vi "INIT.vi"(8 "error in (no error)":errorcluster, 11 "Control-Server in":refnum<class "Control-Server.lvclass">) -> (0 "error out":errorcluster, 3 "Control-Server out":refnum<class "Control-Server.lvclass">)   [LabVIEW 2018, in "Control-Server.lvclass"]
uses:
  Control-Server.lvclass
  Config/config_names_def.ctl
  Config/Config.lvclass
  Control-Server.lvclass/Control-Server.ctl
  dependecies/globalVarII.vi
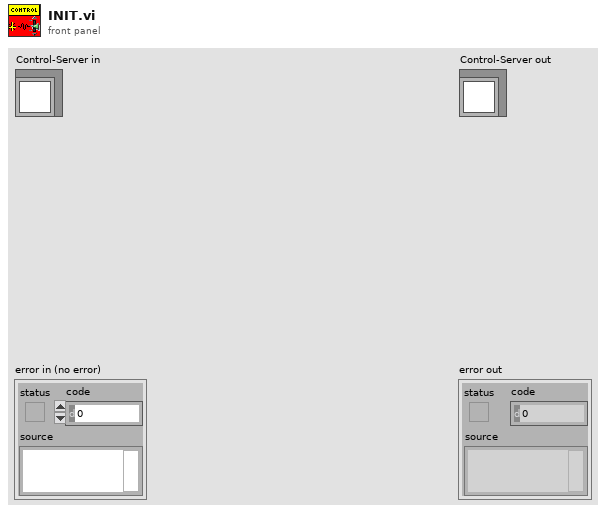
[diagram p1: front panel]
types:
  T1 = typedef "Config.lvclass/config_names_def.ctl" = string
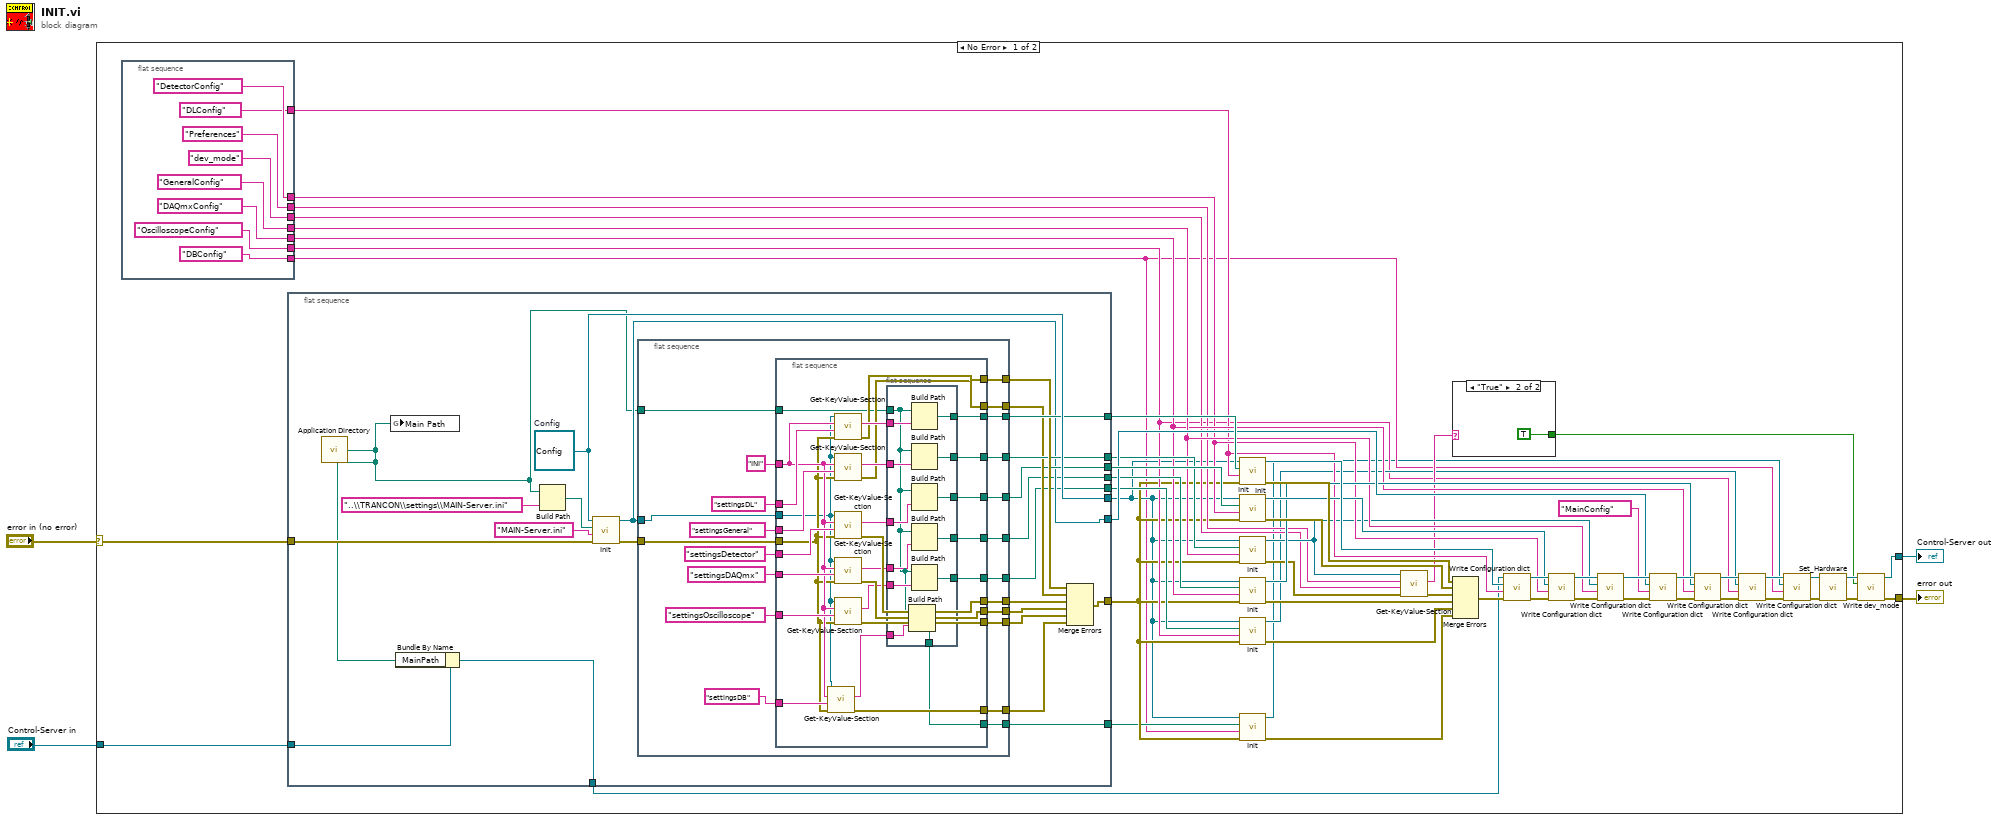
[diagram p0: block diagram]
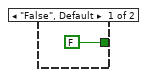
[diagram p2: hidden frame]
diagram:
  n1 = case shown="No Error" "error in (no error)" {
    selector: "error in (no error)" -> [w56 w157]
    tunnel: [w23 w157] -> w3
    tunnel: [w24 w156] -> w4
    tunnel: "Control-Server in" -> [w6 w156]
    frame No Error {
      n2 = flat-sequence {
        tunnel: [T1 "GeneralConfig" ("Combo Box")] -> w38
        tunnel: [T1 "DAQmxConfig" ("Combo Box")] -> w37
        tunnel: [T1 "DetectorConfig" ("Combo Box")] -> w36
        tunnel: [T1 "DLConfig" ("Combo Box")] -> w35
        tunnel: ["Preferences" ("Section")] -> w28
        tunnel: ["dev_mode" ("Key")] -> w27
        tunnel: [T1 "OscilloscopeConfig" ("Combo Box")] -> w18
        tunnel: [T1 "DBConfig" ("Combo Box")] -> w8
        frame #0 {
        }
      }
      n3 = flat-sequence {
        tunnel: [w91] -> w10
        tunnel: [w88] -> w57
        tunnel: [w86] -> w42
        tunnel: w56 -> [w82]
        tunnel: [w81] -> w12
        tunnel: [w80] -> w55
        tunnel: [w79] -> w45
        tunnel: [w77] -> w41
        tunnel: [w76] -> w21
        tunnel: [w73] -> w9
        tunnel: w6 -> [w72]
        tunnel: [w70] -> w5
        frame #0 {
          w91 = refnum<class "Config.lvclass"> refnum  # Config
          n4 = call <vilib>:"Application Directory.vi"() -> ("Application Directory"=w71:path)
          n5 = global write "globalVarII.vi" "Main Path"(w71) -> ()
          n6 = Bundle By Name(cluster=w72, "MainPath"=w71) -> (w70:refnum<class "Control-Server.lvclass">)
          n7 = Build Path(base path=w71, name or relative path="..\\TRANCON\\settings\\MAIN-Server.ini" ("nom ou chemin relatif")) -> (appended path=w90:path)
          n8 = call "Init.vi"("error in"=w82, "Name"="MAIN-Server.ini", "Path"=w90, "Config in"=w91) -> ("error out"=w85:errorcluster, "Config out"=w79:refnum<class "Config.lvclass">)  [unwired: 6 in]
          n9 = flat-sequence {
            tunnel: [w113] -> w88
            tunnel: [w111] -> w87
            tunnel: [w110] -> w86
            tunnel: w79 -> [w109]
            tunnel: w85 -> [w106]
            tunnel: [w105] -> w84
            tunnel: [w104] -> w83
            tunnel: w71 -> [w103]
            tunnel: [w102] -> w80
            tunnel: [w100] -> w78
            tunnel: [w99] -> w77
            tunnel: [w97] -> w76
            tunnel: [w96] -> w75
            tunnel: [w94] -> w74
            tunnel: [w93] -> w73
            frame #0 {
              n10 = flat-sequence {
                tunnel: "settingsDL" ("Key") -> [w142]
                tunnel: [w140] -> w113
                tunnel: "settingsGeneral" ("Key") -> [w139]
                tunnel: [w138] -> w111
                tunnel: [w136] -> w110
                tunnel: w109 -> [w116]
                tunnel: "INI" ("Section") -> [w120]
                tunnel: "settingsDetector" ("Key") -> [w135]
                tunnel: w106 -> [w118]
                tunnel: [w134] -> w105
                tunnel: [w133] -> w104
                tunnel: w103 -> [w127]
                tunnel: [w131] -> w102
                tunnel: "settingsDAQmx" ("Key") -> [w130]
                tunnel: [w129] -> w100
                tunnel: [w126] -> w99
                tunnel: "settingsOscilloscope" ("Key") -> [w125]
                tunnel: [w123] -> w97
                tunnel: [w122] -> w96
                tunnel: "settingsDB" ("Key") -> [w121]
                tunnel: [w117] -> w94
                tunnel: [w115] -> w93
                frame #0 {
                  n11 = call-dynamic "Get-KeyValue-Section.vi"("error in (no error)"=w118, "Key"=w121, "Section"=w120, "Config in"=w116) -> ("error out"=w117:errorcluster, "Value"=w119:string)  [unwired: 5 in, 1 out]
                  n12 = call-dynamic "Get-KeyValue-Section.vi"("error in (no error)"=w118, "Key"=w142, "Section"=w120, "Config in"=w116) -> ("error out"=w138:errorcluster, "Value"=w141:string)  [unwired: 5 in, 1 out]
                  n13 = call-dynamic "Get-KeyValue-Section.vi"("error in (no error)"=w118, "Key"=w139, "Section"=w120, "Config in"=w116) -> ("error out"=w134:errorcluster, "Value"=w137:string)  [unwired: 5 in, 1 out]
                  n14 = call-dynamic "Get-KeyValue-Section.vi"("error in (no error)"=w118, "Key"=w135, "Section"=w120, "Config in"=w116) -> ("error out"=w133:errorcluster, "Value"=w132:string)  [unwired: 5 in, 1 out]
                  n15 = call-dynamic "Get-KeyValue-Section.vi"("error in (no error)"=w118, "Key"=w130, "Section"=w120, "Config in"=w116) -> ("error out"=w129:errorcluster, "Value"=w128:string)  [unwired: 5 in, 1 out]
                  n16 = call-dynamic "Get-KeyValue-Section.vi"("error in (no error)"=w118, "Key"=w125, "Section"=w120, "Config in"=w116) -> ("error out"=w122:errorcluster, "Value"=w124:string)  [unwired: 5 in, 1 out]
                  n17 = flat-sequence {
                    tunnel: w141 -> [w155]
                    tunnel: [w154] -> w140
                    tunnel: w137 -> [w153]
                    tunnel: [w152] -> w136
                    tunnel: w132 -> [w151]
                    tunnel: [w150] -> w131
                    tunnel: w128 -> [w149]
                    tunnel: w127 -> [w144]
                    tunnel: [w148] -> w126
                    tunnel: w124 -> [w147]
                    tunnel: [w146] -> w123
                    tunnel: w119 -> [w145]
                    tunnel: [w143] -> w115
                    frame #0 {
                      n18 = Build Path(base path=w144, name or relative path=w145) -> (appended path=w143:path)
                      n19 = Build Path(base path=w144, name or relative path=w155) -> (appended path=w154:path)
                      n20 = Build Path(base path=w144, name or relative path=w153) -> (appended path=w152:path)
                      n21 = Build Path(base path=w144, name or relative path=w151) -> (appended path=w150:path)
                      n22 = Build Path(base path=w144, name or relative path=w149) -> (appended path=w148:path)
                      n23 = Build Path(base path=w144, name or relative path=w147) -> (appended path=w146:path)
                    }
                  }
                }
              }
            }
          }
          n24 = Merge Errors(w87, w84, w83, w78, w75, w74) -> (w81:errorcluster)
        }
      }
      n25 = call "Init.vi"("error in"=w12, "Name"=w35, "Path"=w57, "Config in"=w10) -> ("error out"=w59:errorcluster, "Config out"=w54:refnum<class "Config.lvclass">)  [unwired: 6 in]
      n26 = call "Init.vi"("error in"=w12, "Name"=w36, "Path"=w55, "Config in"=w10) -> ("error out"=w58:errorcluster, "Config out"=w51:refnum<class "Config.lvclass">)  [unwired: 6 in]
      n27 = call "Init.vi"("error in"=w12, "Name"=w38, "Path"=w42, "Config in"=w10) -> ("error out"=w31:errorcluster, "Config out"=w29:refnum<class "Config.lvclass">)  [unwired: 6 in]
      n28 = call "Init.vi"("error in"=w12, "Name"=w37, "Path"=w41, "Config in"=w10) -> ("error out"=w39:errorcluster, "Config out"=w40:refnum<class "Config.lvclass">)  [unwired: 6 in]
      n29 = call "Init.vi"("error in"=w12, "Name"=w18, "Path"=w21, "Config in"=w10) -> ("error out"=w22:errorcluster, "Config out"=w19:refnum<class "Config.lvclass">)  [unwired: 6 in]
      n30 = call "Init.vi"("error in"=w12, "Name"=w8, "Path"=w9, "Config in"=w10) -> ("error out"=w11:errorcluster, "Config out"=w7:refnum<class "Config.lvclass">)  [unwired: 6 in]
      n31 = call-dynamic "Get-KeyValue-Section.vi"("error in (no error)"=w31, "Key"=w27, "Section"=w28, "Config in"=w29) -> ("error out"=w30:errorcluster, "Value"=w26:string)  [unwired: 5 in, 1 out]
      n32 = case shown="\"True\"" w26 {
        tunnel: [FALSE TRUE] -> w25
        frame "False", Default {
        }
        frame "True" {
        }
      }
      n33 = Merge Errors(w59, w58, w30, w39, w22, w11) -> (w49:errorcluster)
      n34 = call "Write Configuration dict.vi"("error in (no error)"=w49, "Config Name"=w35, "Config.lvclass"=w54, "Control in"=w5) -> ("error out"=w52:errorcluster, "Control out"=w53:refnum<class "Control-Server.lvclass">)  [unwired: 6 in]
      n35 = call "Write Configuration dict.vi"("error in (no error)"=w52, "Config Name"=w36, "Config.lvclass"=w51, "Control in"=w53) -> ("error out"=w48:errorcluster, "Control out"=w50:refnum<class "Control-Server.lvclass">)  [unwired: 6 in]
      n36 = call "Write Configuration dict.vi"("error in (no error)"=w48, "Config Name"=w38, "Config.lvclass"=w29, "Control in"=w50) -> ("error out"=w47:errorcluster, "Control out"=w46:refnum<class "Control-Server.lvclass">)  [unwired: 6 in]
      n37 = call "Write Configuration dict.vi"("error in (no error)"=w47, "Config Name"=T1 "MainConfig" ("Combo Box"), "Config.lvclass"=w45, "Control in"=w46) -> ("error out"=w43:errorcluster, "Control out"=w44:refnum<class "Control-Server.lvclass">)  [unwired: 6 in]
      n38 = call "Write Configuration dict.vi"("error in (no error)"=w43, "Config Name"=w37, "Config.lvclass"=w40, "Control in"=w44) -> ("error out"=w17:errorcluster, "Control out"=w20:refnum<class "Control-Server.lvclass">)  [unwired: 6 in]
      n39 = call "Write Configuration dict.vi"("error in (no error)"=w17, "Config Name"=w18, "Config.lvclass"=w19, "Control in"=w20) -> ("error out"=w16:errorcluster, "Control out"=w13:refnum<class "Control-Server.lvclass">)  [unwired: 6 in]
      n40 = call "Write Configuration dict.vi"("error in (no error)"=w16, "Config Name"=w8, "Config.lvclass"=w7, "Control in"=w13) -> ("error out"=w15:errorcluster, "Control out"=w14:refnum<class "Control-Server.lvclass">)  [unwired: 6 in]
      n41 = call "Set_Hardware.vi"("error in (no error)"=w15, "Control in"=w14) -> ("error out"=w33:errorcluster, "Control out"=w32:refnum<class "Control-Server.lvclass">)  [unwired: 8 in]
      n42 = call-dynamic "Write dev_mode.vi"("error in (no error)"=w33, "dev_mode"=w25, "Control in"=w32) -> ("error out"=w23:errorcluster, "Control out"=w24:refnum<class "Control-Server.lvclass">)  [unwired: 7 in]
    }
    frame Error {
    }
  }
  "error out" <- w3
  "Control-Server out" <- w4
